vi "WRITE_ENET.vi"(4 "error In":errorcluster, 6 "String a ser Enviado":string="*IDN?", 7 "LNA VISA session (for class)":refnum<visa-resource-name>) -> (0 "error out":errorcluster, 1 "String Enviado":string, 3 "LNA VISA session saida":refnum<visa-resource-name>)   [LabVIEW 2018]
uses:
  <vilib>/Instr/_visa.llb/VISA Flush IO Buffer Mask.ctl
panel:
  out "String Lida 2":string
  in  "error in (no error) 2":errorcluster
  out "error out 3":errorcluster
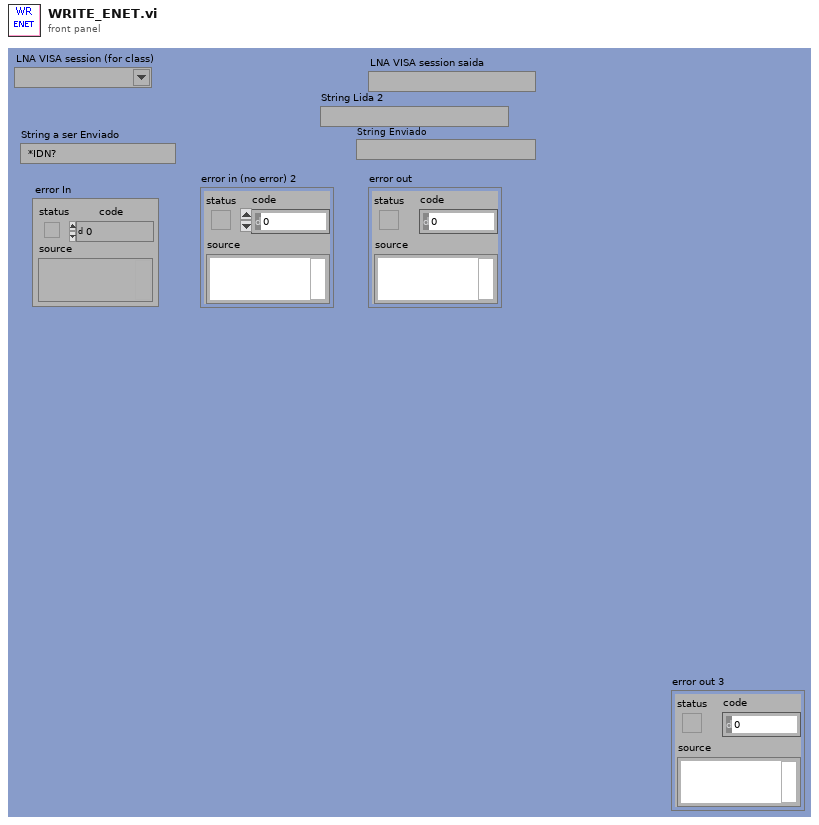
[diagram p1: front panel]
types:
  T1 = typedef "VISA Flush IO Buffer Mask.ctl" = u16
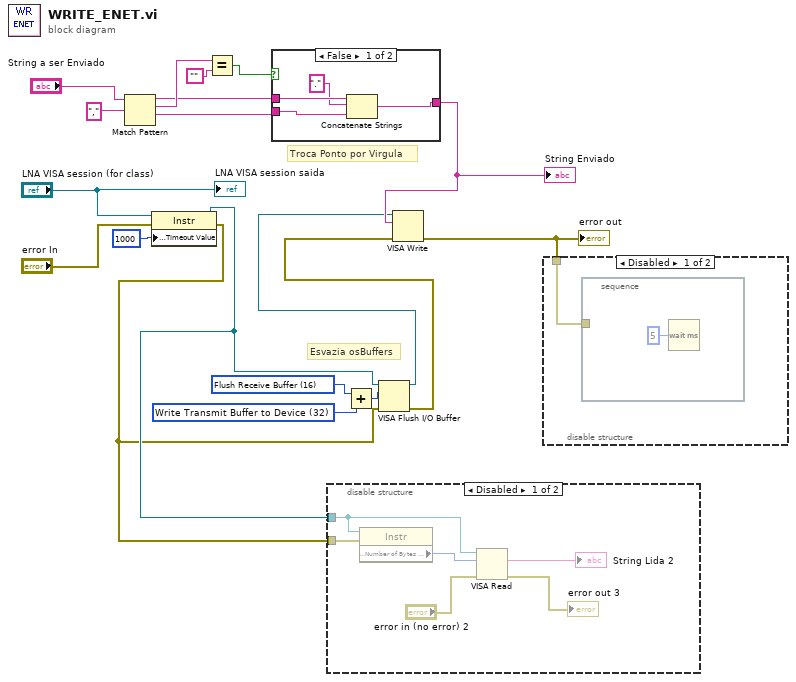
[diagram p0: block diagram]
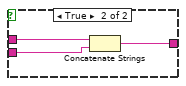
[diagram p4: hidden frame]
diagram:
  w4 = T1 32 items=["Flush Receive Buffer"=16, "Write Transmit Buffer to Device"=32, "Flush Receive Buffer (No I/O)"=64, "Flush Transmit Buffer"=128] ("Mask")
  w5 = T1 16 items=["Flush Receive Buffer"=16, "Write Transmit Buffer to Device"=32, "Flush Receive Buffer (No I/O)"=64, "Flush Transmit Buffer"=128] ("Mask")
  # "Esvazia osBuffers"
  # "Troca Ponto por Virgula"
  n1 = Match Pattern(string="String a ser Enviado", regular expression=",") -> (before substring=w11:string, match substring=w13:string, after substring=w10:string)  [unwired: 1 in, 1 out]
  n2 = property class="Instr"(reference="LNA VISA session (for class)", error in="error In", "General Settings:Timeout Value"=u32 1000 ("Tmo Value")) -> (reference out=w7:refnum<visa-resource-name>, error out=w6:errorcluster)
  n3 = Equal?(x=w13, y="") -> (x = y?=w12:bool)
  n4 = case shown="False" w12 {
    tunnel: [w20 w26] -> w15
    tunnel: w11 -> [w23 w25]
    tunnel: w10 -> [w22 w24]
    frame False {
      n5 = Concatenate Strings(w23, ".", w22) -> (w20:string)
    }
    frame True {
      n6 = Concatenate Strings(w25, w24) -> (w26:string)
    }
  }
  "String Enviado" <- w15
  n7 = disable-structure shown="Disabled" {
    disable-tunnel: w7 -> [w32 _]
    disable-tunnel: w6 -> [w31 _]
    frame Disabled {
      n8 = property class="Instr"(reference=w32, error in=w31) -> ("Serial Settings:Number of Bytes at Serial Port"=w30:u32)  [unwired: 2 out]
      n9 = VISA Read(VISA resource name=w32, byte count=w30, error in (no error)="error in (no error) 2") -> (read buffer=→"String Lida 2":string, error out=→"error out 3":errorcluster)  [unwired: 2 out]
    }
    frame Enabled {
    }
  }
  n10 = Add(x=w5, y=w4) -> (x+y=w3:T1)
  n11 = VISA Flush I/O Buffer(VISA resource name=w7, mask (16)=w3, error in (no error)=w6) -> (VISA resource name out=w2:refnum<visa-resource-name>, error out=w1:errorcluster)
  n12 = VISA Write(VISA resource name=w2, write buffer=w15, error in (no error)=w1) -> (error out=w8:errorcluster)  [unwired: 2 out]
  "error out" <- w8
  n13 = disable-structure shown="Disabled" {
    disable-tunnel: w8 -> [w33 _]
    frame Disabled {
      n14 = stacked-sequence {
        tunnel: w33 -> [_]
        frame #0 {
          n15 = Wait (ms)(milliseconds to wait=u32 5) -> ()  [unwired: 1 out]
        }
      }
    }
    frame Enabled {
    }
  }
  "LNA VISA session saida" <- "LNA VISA session (for class)"
